vi "GT_CrdStart.vi"(3 "fifo in":i16, 4 "crd in":i16, 5 "rtn_In":cluster{"rtn":i16, "Func":string}) -> (0 "fifo out":i16, 1 "crd out":i16, 2 "rtn_Out":cluster{"rtn":i16, "Func":string})   [LabVIEW 2014]
uses:
  axxon_Gold.vi
  VC6/gts.dll
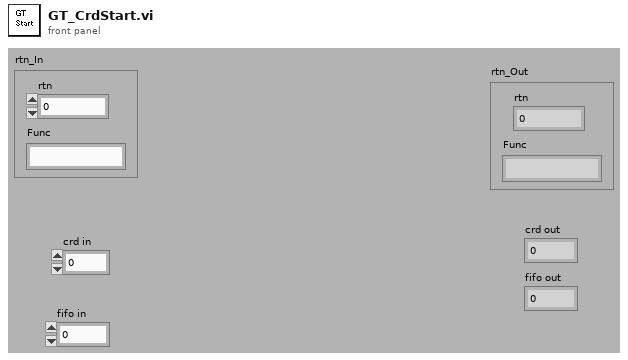
[diagram p1: front panel]
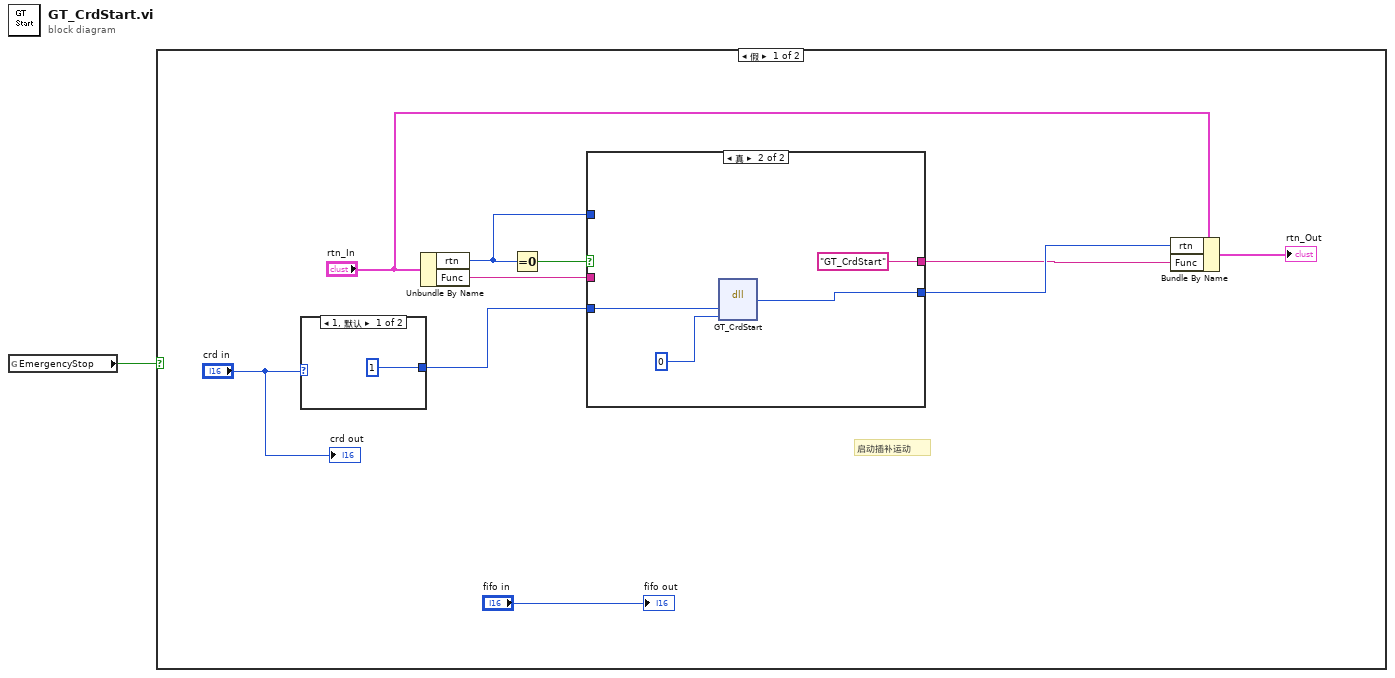
[diagram p0: block diagram]
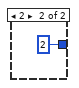
[diagram p2: hidden frame]
diagram:
  n1 = global read "axxon_Gold.vi" "EmergencyStop"() -> (w1:bool)
  n2 = case shown="假" w1 {
    frame False {
      # "启动插补运动"
      n3 = case shown="1, 默认" "crd in" {
        tunnel: [i16 1 ("mask") i16 2 ("mask")] -> w3
        frame 1, Default {
        }
        frame 2 {
        }
      }
      n4 = Unbundle By Name("rtn_In") -> ("rtn"=w5:i16, "Func"=w6:string)
      n5 = Equal To 0?(x=w5) -> (x = 0?=w11:bool)
      n6 = case shown="真" w11 {
        tunnel: [w14 w19] -> w8
        tunnel: [w15 "GT_CrdStart" ("Func")] -> w7
        tunnel: w3 -> [_ w17]
        tunnel: w6 -> [w15 _]
        tunnel: w5 -> [w14 _]
        frame False {
        }
        frame True {
          n7 = dll-call lib="PTH2Fabs DNewGTS AC-800LWin7版源程序-20170926gts85VC6gts.dll" fn="GT_CrdStart"("mask"=w17, "option"=i16 0) -> ("rtn"=w19:i16)  [unwired: 5 in, 2 out]
        }
      }
      n8 = Bundle By Name(cluster="rtn_In", "rtn"=w8, "Func"=w7) -> (→"rtn_Out":cluster{"rtn":i16, "Func":string})
      "crd out" <- "crd in"
      "fifo out" <- "fifo in"
    }
    frame True {
    }
  }
